vi "NUWARRunMATLABProg.vi"(6 "Program Control":T2, 7 "SampleRate":i32, 8 "Load Prog Exported from MATALB":bool, 9 "Device Number i32 (0)":i32 min=0) -> (0 "Program Summary":T1, 1 "Program Loaded":bool, 2 "Initializing":bool, 3 "ProgReady":bool)   [LabVIEW 2020]
panel:
  in  "InitState":i32
  in  "First Pos":string
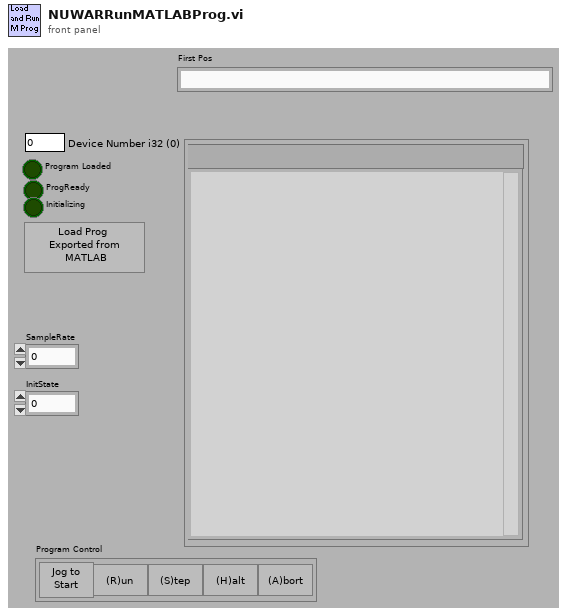
[diagram p1: front panel]
types:
  T1 = cluster{"Output Path (NotAPath if cancelled)":path, "String 3":string}
  T2 = cluster{"Start Program":bool, "Abort Program":bool, "Step Program":bool, "Halt Program":bool, "Jog To Start":bool}
  T3 = cluster{"Coord Number i32 (1-8) (1)":i32, "Motor Number i32 (1-8) (1)":i32, "Convert  Bool":bool}
  T4 = cluster{"Output Path (NotAPath if cancelled)":path, string}
  T5 = cluster{"Program Loaded":bool, "Program Number i32":i32, "Coord Number i32":i32}
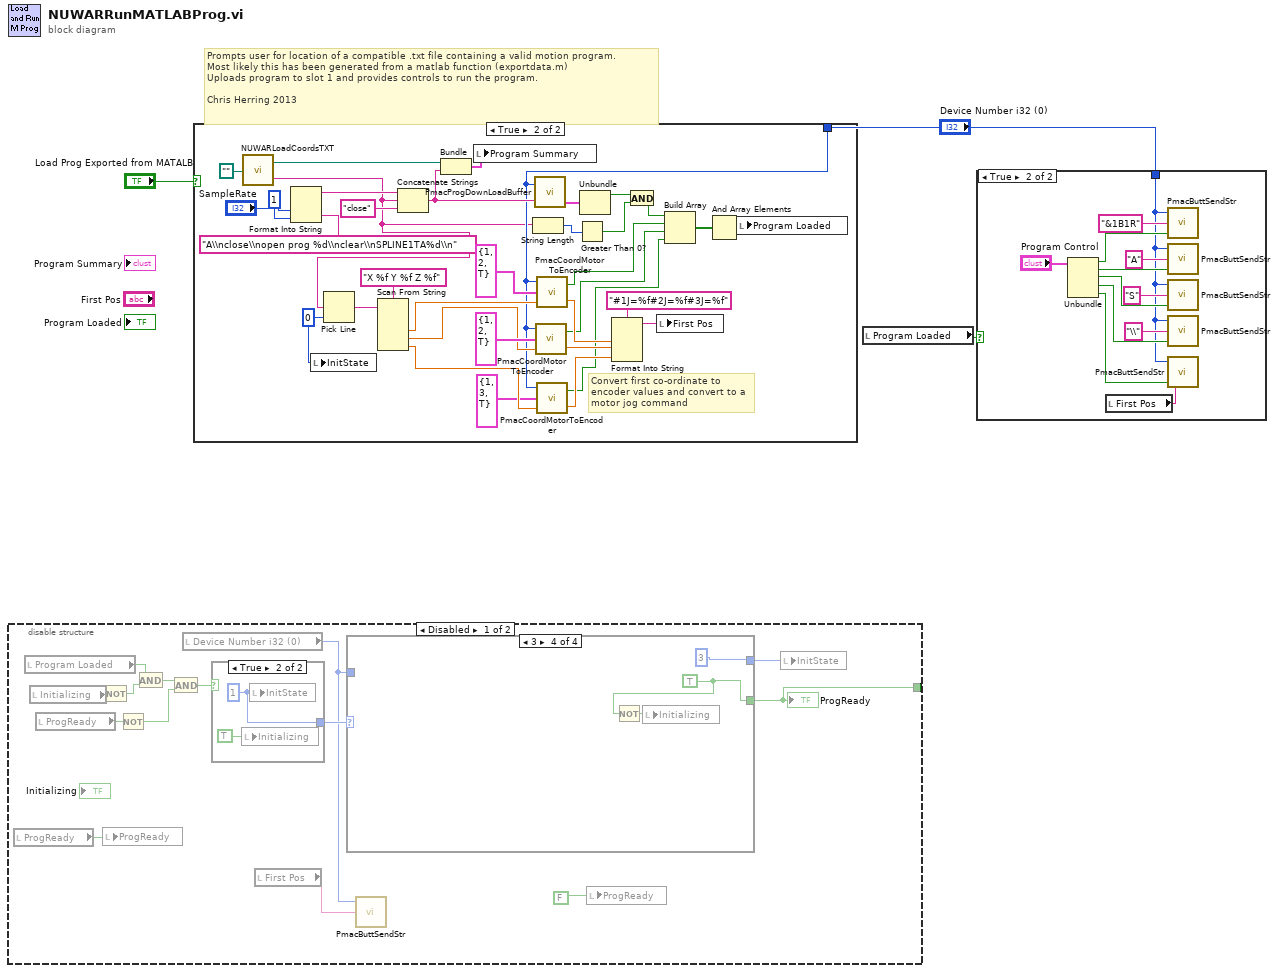
[diagram p0: block diagram]
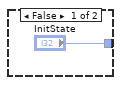
[diagram p2: hidden frame]
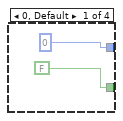
[diagram p3: hidden frame]
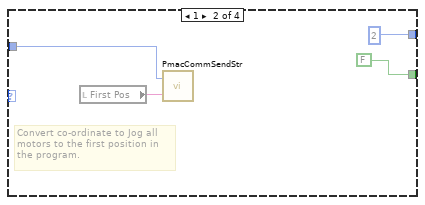
[diagram p4: hidden frame]
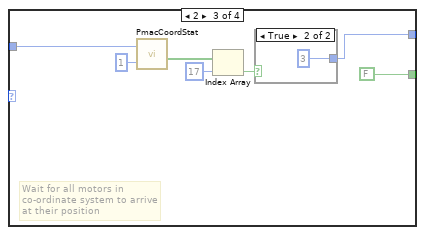
[diagram p5: hidden frame]
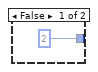
[diagram p6: hidden frame]
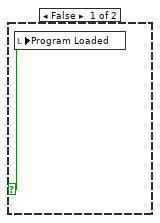
[diagram p8: hidden frame]
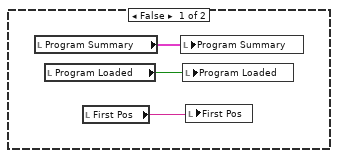
[diagram p9: hidden frame]
diagram:
  # "Prompts user for location of a compatible .txt file containing a valid motion program.\nMost likely this has been generated from a matlab function (exportdata.m)\nUploads program to slot 1 and provides controls to run the program.\n\nChris Herring 2013"
  n1 = disable-structure shown="Disabled" {
    disable-tunnel: [w9 _] -> _
    frame Disabled {
      n2 = local read "ProgReady"() -> (w5:bool)
      n3 = local read "Program Loaded"() -> (w18:bool)
      n4 = local read "Initializing"() -> (w11:bool)
      n5 = local read "ProgReady"() -> (w12:bool)
      n6 = Not(x=w11) -> (.not. x?=w14:bool)
      n7 = local write "ProgReady"(w5) -> ()
      n8 = Not(x=w12) -> (.not. x?=w13:bool)
      n9 = And(x=w18, y=w14) -> (x .and. y?=w15:bool)
      n10 = And(x=w15, y=w13) -> (x .and. y?=w16:bool)
      n11 = local read "Device Number i32 (0)"() -> (w6:i32)
      n12 = case shown="True" w16 {
        tunnel: ["InitState" w21] -> w17
        frame False {
        }
        frame True {
          w21 = 1 ("InitState")
          n13 = local write "Initializing"(TRUE ("Initializing")) -> ()
          n14 = local write "InitState"(w21) -> ()
        }
      }
      n15 = local read "First Pos"() -> (w7:string)
      n16 = case shown="3" w17 {
        tunnel: w6 -> [_ w27 w34 _]
        tunnel: [FALSE ("Ready") FALSE ("Ready") FALSE ("Ready") w37] -> w9
        tunnel: [0 ("InitState") 2 ("InitState") w28 3 ("InitState")] -> w10
        frame 0, Default {
        }
        frame 1 {
          # "Convert co-ordinate to Jog all motors to the first position in the program."
          n17 = local read "First Pos"() -> (w26:string)
          n18 = call "PmacCommSendStr.vi"("Command String"=w26, "Device Number i32 (0)"=w27) -> ()  [unwired: 1 out]
        }
        frame 2 {
          # "Wait for all motors in co-ordinate system to arrive at their position"
          n19 = call "PmacCoordStat.vi"("Device Number i32 (0)"=w34, "Coord Number i32 (1-8) (1)"=1) -> ("Second Word 24 Element Bool Array"=w32:bool[])  [unwired: 3 out]
          n20 = Index Array(array=w32, index=17) -> (element=w30:bool)
          n21 = case shown="True" w30 {
            tunnel: [2 ("InitState") 3 ("InitState")] -> w28
            frame False {
            }
            frame True {
            }
          }
        }
        frame 3 {
          w37 = TRUE ("Ready")
          n22 = Not(x=w37) -> (.not. x?=w39:bool)
          n23 = local write "Initializing"(w39) -> ()
        }
      }
      "ProgReady" <- w9
      n24 = call "PmacButtSendStr.vi"("Command String"=w7, "Device Number i32 (0)"=w6) -> ("Button State Bool"=w8:bool)  [unwired: 1 out]
      n25 = local write "ProgReady"(FALSE ("Ready")) -> ()
      n26 = local write "InitState"(w10) -> ()
    }
    frame Enabled {
    }
  }
  n27 = case shown="True" "Load Prog Exported from MATALB" {
    tunnel: "Device Number i32 (0)" -> [_ w58]
    frame False {
      n28 = local read "Program Summary"() -> (w42:T1)
      n29 = local read "Program Loaded"() -> (w41:bool)
      n30 = local read "First Pos"() -> (w40:string)
      n31 = local write "Program Summary"(w42) -> ()
      n32 = local write "Program Loaded"(w41) -> ()
      n33 = local write "First Pos"(w40) -> ()
    }
    frame True {
      w44 = 0 ("line index")
      # "Convert first co-ordinate to encoder values and convert to a motor jog command"
      n34 = call "NUWARLoadCoordsTXT.vi"("Input Path (dialog if empty)"=path "") -> ("Output Path (NotAPath if cancelled)"=w72:path, "Buffer String"=w51:string)
      n35 = Format Into String(format string="A\\nclose\\nopen prog %d\\nclear\\nSPLINE1TA%d\\n" ("String 3"), 1, "SampleRate") -> (resulting string=w74:string)  [unwired: 2 in, 1 out]
      n36 = local write "InitState"(w44) -> ()
      n37 = Pick Line(multi-line string=w51, line index=w44) -> (output string=w52:string)  [unwired: 1 out]
      n38 = Scan From String(format string="X %f Y %f Z %f", input string=w52) -> (output 1=w62:dbl, output 2=w61:dbl, output 3=w60:dbl)  [unwired: 2 in, 6 out]
      n39 = Concatenate Strings(w74, w51, "close" ("string")) -> (w67:string)
      n40 = Bundle("Output Path (NotAPath if cancelled)"=w72, w67) -> (w66:T4)  [unwired: 1 out]
      n41 = local write "Program Summary"(w66) -> ()
      n42 = String Length(string=w51) -> (length=w70:i32)
      n43 = call "PmacProgDownLoadBuffer.vi"("DeviceNumber i32 (0)"=w58, "Program Buffer String"=w67) -> ("Program VI State Cluster"=w71:T5)  [unwired: 2 out]
      n44 = call "PmacCoordMotorToEncoder.vi"("Input Value Double"=w61, "Coord Specify Cluster"=T3 {"Coord Number i32 (1-8) (1)"=1, "Motor Number i32 (1-8) (1)"=2, "Convert  Bool"=TRUE}, "Device Number i32 (0)"=w58) -> ("Output Value Double"=w56:dbl, "Coord Defined Bool"=w46:bool)
      n45 = call "PmacCoordMotorToEncoder.vi"("Input Value Double"=w62, "Coord Specify Cluster"=T3 {"Coord Number i32 (1-8) (1)"=1, "Motor Number i32 (1-8) (1)"=2, "Convert  Bool"=TRUE}, "Device Number i32 (0)"=w58) -> ("Output Value Double"=w57:dbl, "Coord Defined Bool"=w47:bool)
      n46 = call "PmacCoordMotorToEncoder.vi"("Input Value Double"=w60, "Coord Specify Cluster"=T3 {"Coord Number i32 (1-8) (1)"=1, "Motor Number i32 (1-8) (1)"=3, "Convert  Bool"=TRUE}, "Device Number i32 (0)"=w58) -> ("Output Value Double"=w55:dbl, "Coord Defined Bool"=w45:bool)
      n47 = Greater Than 0?(x=w70) -> (x > 0?=w68:bool)
      n48 = Unbundle(w71) -> ("Program Loaded"=w69:bool)  [unwired: 2 out]
      n49 = Format Into String(format string="#1J=%f#2J=%f#3J=%f", w57, w56, w55) -> (resulting string=w53:string)  [unwired: 2 in, 1 out]
      n50 = And(x=w69, y=w68) -> (x .and. y?=w49:bool)
      n51 = local write "First Pos"(w53) -> ()
      n52 = Build Array(w49, w47, w46, w45) -> (w48:bool[])
      n53 = And Array Elements(Boolean array=w48) -> (logical AND=w50:bool)
      n54 = local write "Program Loaded"(w50) -> ()
    }
  }
  n55 = local read "Program Loaded"() -> (w1:bool)
  n56 = case shown="True" w1 {
    selector: w1 -> [w78 _]
    tunnel: "Device Number i32 (0)" -> [_ w81]
    frame False {
      n57 = local write "Program Loaded"(w78) -> ()
    }
    frame True {
      n58 = Unbundle("Program Control") -> ("Start Program"=w89:bool, "Abort Program"=w87:bool, "Step Program"=w84:bool, "Halt Program"=w83:bool, "Jog To Start"=w79:bool)
      n59 = local read "First Pos"() -> (w80:string)
      n60 = call "PmacButtSendStr.vi"("Button State Bool"=w89, "Command String"="&1B1R", "Device Number i32 (0)"=w81) -> ()  [unwired: 1 out]
      n61 = call "PmacButtSendStr.vi"("Button State Bool"=w87, "Command String"="A", "Device Number i32 (0)"=w81) -> ()  [unwired: 1 out]
      n62 = call "PmacButtSendStr.vi"("Button State Bool"=w84, "Command String"="S", "Device Number i32 (0)"=w81) -> ()  [unwired: 1 out]
      n63 = call "PmacButtSendStr.vi"("Button State Bool"=w83, "Command String"="\\", "Device Number i32 (0)"=w81) -> ()  [unwired: 1 out]
      n64 = call "PmacButtSendStr.vi"("Button State Bool"=w79, "Command String"=w80, "Device Number i32 (0)"=w81) -> ()  [unwired: 1 out]
    }
  }
